vi "SetPath.vi"(8 "error in (no error)":errorcluster, 10 "Path":path, 11 "Image in":refnum<class "Image.lvclass">) -> (0 "error out":errorcluster, 3 "Image out":refnum<class "Image.lvclass">)   [LabVIEW 2021, in "Markdown.lvlib" / "Image.lvclass"]
uses:
  Image.lvclass
  Image.lvclass/Image.ctl
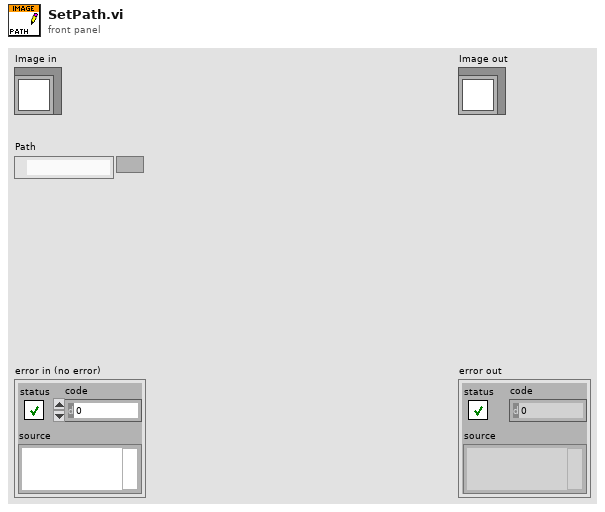
[diagram p1: front panel]
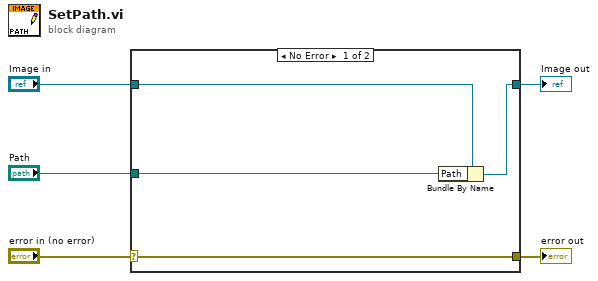
[diagram p0: block diagram]
diagram:
  n1 = case shown="No Error" "error in (no error)" {
    selector: "error in (no error)" -> [w9 w10]
    tunnel: [w9 w10] -> w4
    tunnel: [w7 w11] -> w2
    tunnel: "Image in" -> [w8 w11]
    tunnel: "Path" -> [w6 _]
    frame No Error {
      n2 = Bundle By Name(cluster=w8, "Path"=w6) -> (w7:refnum<class "Image.lvclass">)
    }
    frame Error {
    }
  }
  "error out" <- w4
  "Image out" <- w2
